vi "Fuel Injector Default Section.vi"(8 "error in (no error)":errorcluster, 11 "Node Ptr":T1 format="%.0x") -> (0 "error out":errorcluster)   [LabVIEW 2019, in "Fuel Injector Analysis Addon System Explorer.lvlib"]
uses:
  Fuel Injector Analysis Addon System Explorer.lvlib
  <vilib>/NI VeriStand/Custom Device API/Custom Device Item Ref.ctl
  <vilib>/NI VeriStand/Custom Device API/Custom Device API.lvlib
panel:
  in  "SHDocVw.IWebBrowser":refnum<k7>(container)
  in  "Header":cluster{"Section Name":string}={"Section Name"="Custom Device Item Settings"}
  in  "Description":string
  out "Name":string
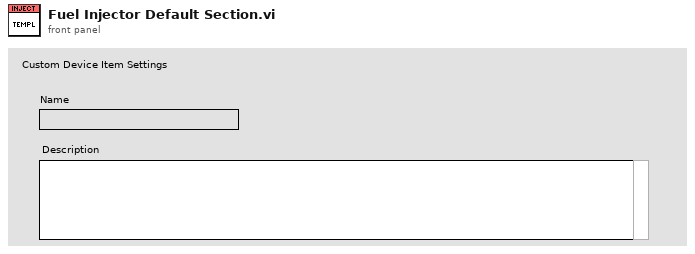
[diagram p1: front panel]
types:
  T1 = typedef "Custom Device API.lvlib/Custom Device Item Ref.ctl" = u64
  T2 = typedef "Custom Device API.lvlib/Custom Device Item Info.ctl" = cluster{"Name":string, "Is Channel":bool, "GUID":string, "Is Waveform":bool}
  T3 = typedef "Custom Device API.lvlib/Custom Device Commands.ctl" = enum16{"Default", "Item renamed", "Shutdown", "Dynamic button pressed"}
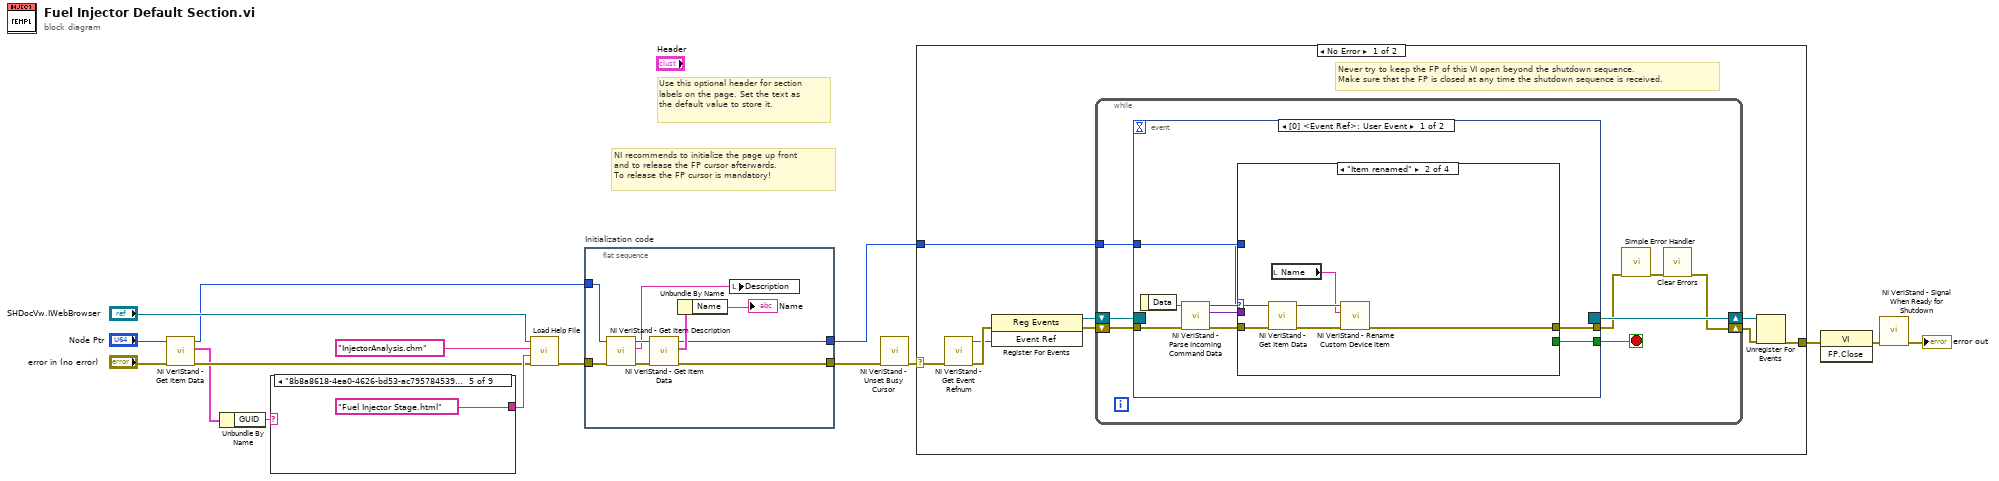
[diagram p0: block diagram]
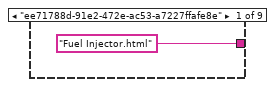
[diagram p2: hidden frame]
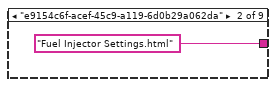
[diagram p3: hidden frame]
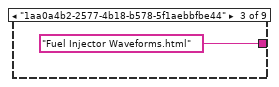
[diagram p4: hidden frame]
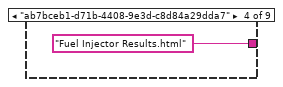
[diagram p5: hidden frame]
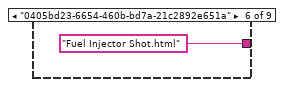
[diagram p6: hidden frame]
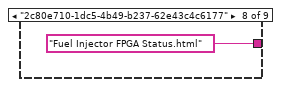
[diagram p8: hidden frame]
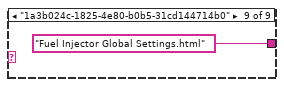
[diagram p9: hidden frame]
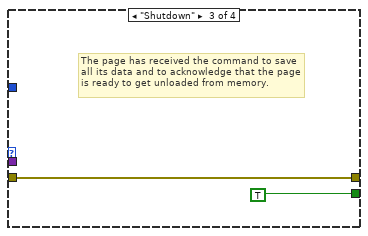
[diagram p11: hidden frame]
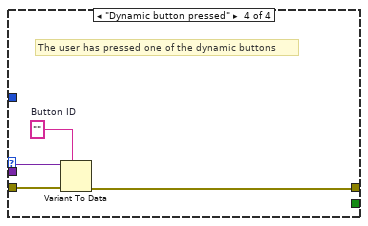
[diagram p12: hidden frame]
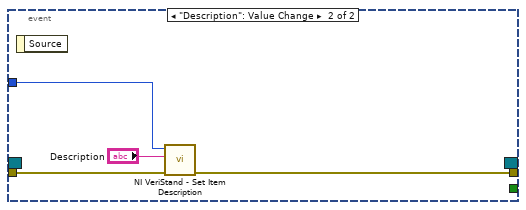
[diagram p13: hidden frame]
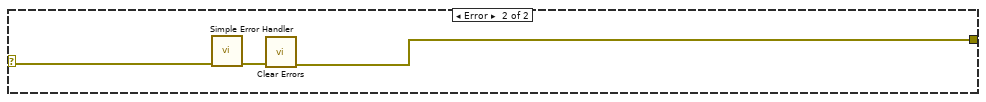
[diagram p14: hidden frame]
diagram:
  # "Use this optional header for section labels on the page. Set the text as the default value to store it."
  # "NI recommends to initialize the page up front\nand to release the FP cursor afterwards.\nTo release the FP cursor is mandatory!"
  n1 = call <vilib>:"NI VeriStand - Get Item Data.vi"("error in (no error)"="error in (no error)", "Item Ref in"="Node Ptr") -> ("error out"=w5:errorcluster, "Item Info"=w2:T2, "Item Ref out"=w3:T1)  [unwired: 7 out]
  n2 = Unbundle By Name(w2) -> ("GUID"=w1:string)
  n3 = case shown="\"8b8a8618-4ea0-4626-bd53-ac7957845392\"" w1 {
    tunnel: ["Fuel Injector.html" ("HTML File") "Fuel Injector Settings.html" ("HTML File") "Fuel Injector Waveforms.html" ("HTML File") "Fuel Injector Results.html" ("HTML File") "Fuel Injector Stage.html" ("HTML File") "Fuel Injector Shot.html" ("HTML File") _ "Fuel Injector FPGA Status.html" ("HTML File") "Fuel Injector Global Settings.html" ("HTML File")] -> w10
    frame "ee71788d-91e2-472e-ac53-a7227ffafe8e" {
    }
    frame "e9154c6f-acef-45c9-a119-6d0b29a062da" {
    }
    frame "1aa0a4b2-2577-4b18-b578-5f1aebbfbe44" {
    }
    frame "ab7bceb1-d71b-4408-9e3d-c8d84a29dda7" {
    }
    frame "8b8a8618-4ea0-4626-bd53-ac7957845392" {
    }
    frame "0405bd23-6654-460b-bd7a-21c2892e651a" {
    }
    frame Default {
    }
    frame "2c80e710-1dc5-4b49-b237-62e43c4c6177" {
    }
    frame "1a3b024c-1825-4e80-b0b5-31cd144714b0" {
    }
  }
  n4 = call "Load Help File.vi"("error in (no error)"=w5, "HTML File"=w10, "Main CHM File"="InjectorAnalysis.chm", "SHDocVw.IWebBrowser2"="SHDocVw.IWebBrowser") -> ("error out"=w7:errorcluster)  [unwired: 7 in]
  n5 = flat-sequence "Initialization code" {
    tunnel: w7 -> [w32]
    tunnel: [w27] -> w13
    tunnel: [w28] -> w11
    tunnel: w3 -> [w25]
    frame #0 {
      n6 = call <vilib>:"NI VeriStand - Get Item Description.vi"("error in (no error)"=w32, "Item Ref in"=w25) -> ("error out"=w30:errorcluster, "Description"=w31:string, "Item Ref out"=w33:T1)  [unwired: 7 out]
      n7 = call <vilib>:"NI VeriStand - Get Item Data.vi"("error in (no error)"=w30, "Item Ref in"=w33) -> ("error out"=w27:errorcluster, "Item Info"=w29:T2, "Item Ref out"=w28:T1)  [unwired: 7 out]
      n8 = Unbundle By Name(w29) -> ("Name"=→"Name":string)
      n9 = local write "Description"(w31) -> ()
    }
  }
  n10 = call <vilib>:"NI VeriStand - Unset Busy Cursor.vi"("error in (no error)"=w13) -> ("error out"=w12:errorcluster)  [unwired: 10 out]
  n11 = case shown="No Error" w12 {
    selector: w12 -> [w34 w78]
    tunnel: [w39 w76] -> w16
    tunnel: w11 -> [w35 _]
    frame No Error {
      # "Never try to keep the FP of this VI open beyond the shutdown sequence.\nMake sure that the FP is closed at any time the shutdown sequence is received."
      n12 = call <vilib>:"NI VeriStand - Get Event Refnum.vi"("error in (no error)"=w34) -> ("error out"=w42:errorcluster, "Event Ref"=w38:refnum<user-event>)  [unwired: 9 out]
      n13 = register-events(error in=w42, w38) -> (reference out=w36:refnum<event-registration>, error out=w37:errorcluster)  [unwired: 1 in]
      n14 = while {
        tunnel: w35 -> [w46]
        shift-right: [w43] -> w40
        shift-left: w37 -> [w49]
        shift-right: [w50] -> w41
        shift-left: w36 -> [w48]
        stop <- w47 stop-if-true
        n15 = event shown="[0] <Event Ref>: User Event" {
          selector: w48 -> [_ _]
          dyn-events: [_ _] -> w50
          timeout: _ -> [_ _]
          tunnel: w49 -> [w58 w74]
          tunnel: [w54 _] -> w47
          tunnel: [w53 w73] -> w45
          tunnel: w46 -> [w52 w75]
          event User Event {
            n16 = event-data() -> ("Data"=w57:string)  [unwired: 1 out]
            n17 = call <vilib>:"NI VeriStand - Parse Incoming Command Data.vi"("error in (no error)"=w58, "Incoming data"=w57) -> ("error out"=w56:errorcluster, "Outgoing data"=w51:variant, "Action"=w55:T3)  [unwired: 7 out]
            n18 = case shown="\"Item renamed\"" w55 {
              tunnel: w56 -> [w59 w65 w66 w71]
              tunnel: [_ _ TRUE _] -> w54
              tunnel: [w59 w60 w66 w68] -> w53
              tunnel: w52 -> [_ w64 _ _]
              tunnel: w51 -> [_ _ _ w70]
              frame "Default", Default {
              }
              frame "Item renamed" {
                n19 = call <vilib>:"NI VeriStand - Get Item Data.vi"("error in (no error)"=w65, "Item Ref in"=w64) -> ("error out"=w63:errorcluster, "Item Ref out"=w62:T1)  [unwired: 8 out]
                n20 = local read "Name"() -> (w61:string)
                n21 = call <vilib>:"NI VeriStand - Rename Custom Device Item.vi"("error in (no error)"=w63, "New Name"=w61, "Item Ref in"=w62) -> ("error out"=w60:errorcluster)  [unwired: 6 in, 2 out]
              }
              frame "Shutdown" {
                # "The page has received the command to save all its data and to acknowledge that the page is ready to get unloaded from memory."
              }
              frame "Dynamic button pressed" {
                w69 = ""  # Button ID
                # "The user has pressed one of the dynamic buttons"
                n22 = Variant To Data(error in=w71, type=w69, Variant=w70) -> (error out=w68:errorcluster)  [unwired: 1 out]
              }
            }
          }
          event "Description": Value Change {
            n23 = event-data() -> ()  [unwired: 2 out]
            n24 = call <vilib>:"NI VeriStand - Set Item Description.vi"("error in (no error)"=w74, "Description"="Description", "Item Ref in"=w75) -> ("error out"=w73:errorcluster)  [unwired: 8 out]
          }
        }
        n25 = call <vilib>:"Simple Error Handler.vi"("error in (no error)"=w45) -> ("error out"=w44:errorcluster)  [unwired: 1 in, 7 out]
        n26 = call <vilib>:"Clear Errors.vi"("error in (no error)"=w44) -> ("error out"=w43:errorcluster)  [unwired: 1 in, 5 out]
      }
      n27 = Unregister For Events(event registration refnum=w41, error in=w40) -> (error out=w39:errorcluster)
    }
    frame Error {
      n28 = call <vilib>:"Simple Error Handler.vi"("error in (no error)"=w78) -> ("error out"=w77:errorcluster)  [unwired: 1 in, 7 out]
      n29 = call <vilib>:"Clear Errors.vi"("error in (no error)"=w77) -> ("error out"=w76:errorcluster)  [unwired: 1 in, 5 out]
    }
  }
  n30 = invoke class="VI" method="FP.Close"(error in=w16) -> (error out=w15:errorcluster)  [unwired: 2 in, 2 out]
  n31 = call <vilib>:"NI VeriStand - Signal When Ready for Shutdown.vi"("error in (no error)"=w15) -> ("error out"=→"error out":errorcluster)  [unwired: 10 out]
